vi "溶解氧电极校准.vi"() -> ()   [LabVIEW 2016, in "斯坦道多参数.lvlib"]
uses:
  <vilib>/Analysis/NI_AALBase.lvlib
  <vilib>/Utility/miscctls.llb/LVPointTypeDef.ctl
  <vilib>/Plasmionique/MB Master/MB_Master_Serial/MB_Master_Serial.lvclass
  C:/Program Files (x86)/National Instruments/LabVIEW 2016/vi.lib/Plasmionique/MB Master/MB_Master/MB_Master.lvclass
panel:
  out "变异系数":dbl
  out "standard deviation":dbl caption="标准差" format="%0.2f"
  out "mean":dbl caption="均值" format="%0.2f"
  out "测量读值":dbl
  out "偏移值补偿":dbl
  out "当前读值":dbl caption="饱和度值"
  out "提示":string
  in  "第二点通过校正":bool
  in  "第一点通过校正":bool
  in  "饱和度校正":bool
  in  "零点校正":bool
  out "气压补偿值":dbl
  out "盐度补偿值":dbl
  out "电极斜率":dbl
  out "电极零点":dbl
  # "溶解氧电极设定"
  # "%"
  # "ppt"
  # "%"
  # "hPa"
  # "%"
  # "mg/L"
  # "mg/L"
  # "电极校正"
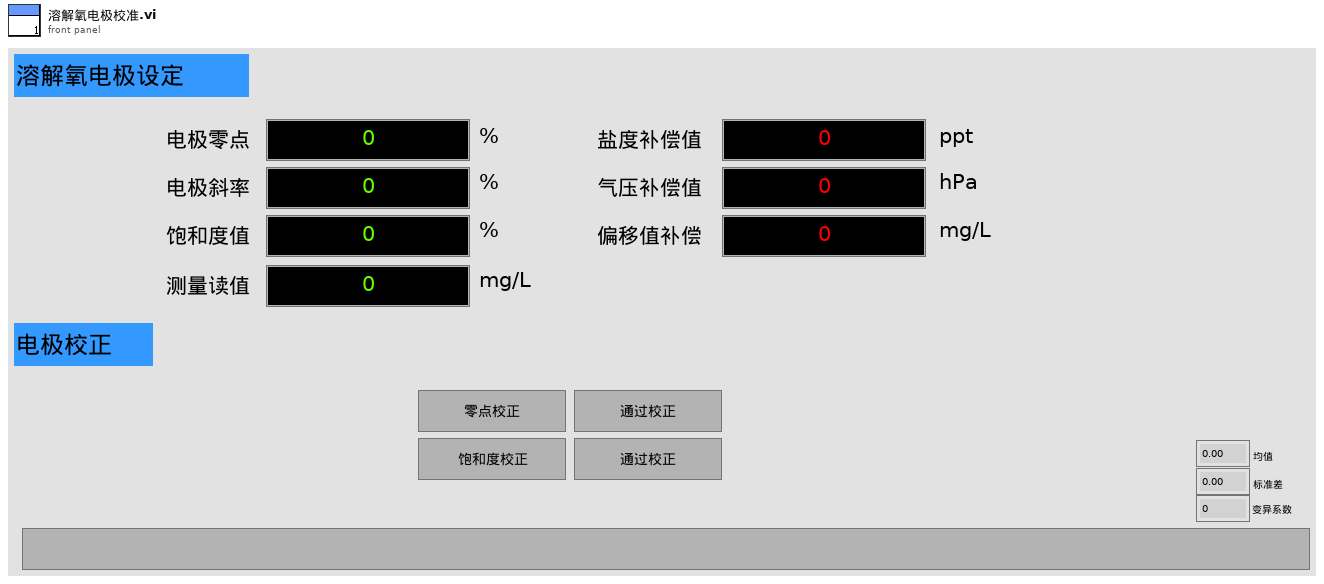
[diagram p1: front panel]
types:
  T1 = typedef "LVPointTypeDef.ctl" = cluster{"Horizontal":i16, "Vertical":i16}
  T2 = typedef "斯坦道多参数.lvlib/校准步骤.ctl" = enum16{"待机", "放置第一点标液", "第一点校准启动", "第一点校准写入", "第一点校准失败", "放置第二点标液", "第二点校准启动", "第二点校准写入", "第二点校准失败", "校准结果写入", "校准结束"}
  T3 = cluster{"电极状态标志":u16, "电极型号标志":u16, "溶解氧测量值":sgl, "温度测量值":sgl, "溶解氧饱和度值":sgl, "盐度补偿值":sgl, "大气压补偿值":sgl, "溶解氧偏移修正值":sgl, "温度偏移修正值":sgl, "手动温度补偿值":sgl, "溶解氧电极零点":sgl, "溶解氧电极斜率":sgl, "第1点标准值记录":sgl, "第1点信号值记录":sgl, "第1点温度值记录":sgl, "第2点标准值记录":sgl, "第2点信号值记录":sgl, "第2点温度值记录":sgl, "命令滤波设定":u16, "温度模式":enum16{"ATC", "MTC"}, "生产批次":u16, "电极序号":u16, "串口地址":u16, "串口波特率":enum16{"9600", "19200", "115200"}, "串口校验位":enum16{"NONE", "ODD", "EVEN"}, "串口停止位":enum16{"1bit", "2bit"}, "第一点标准值":sgl, "第二点标准值":sgl}
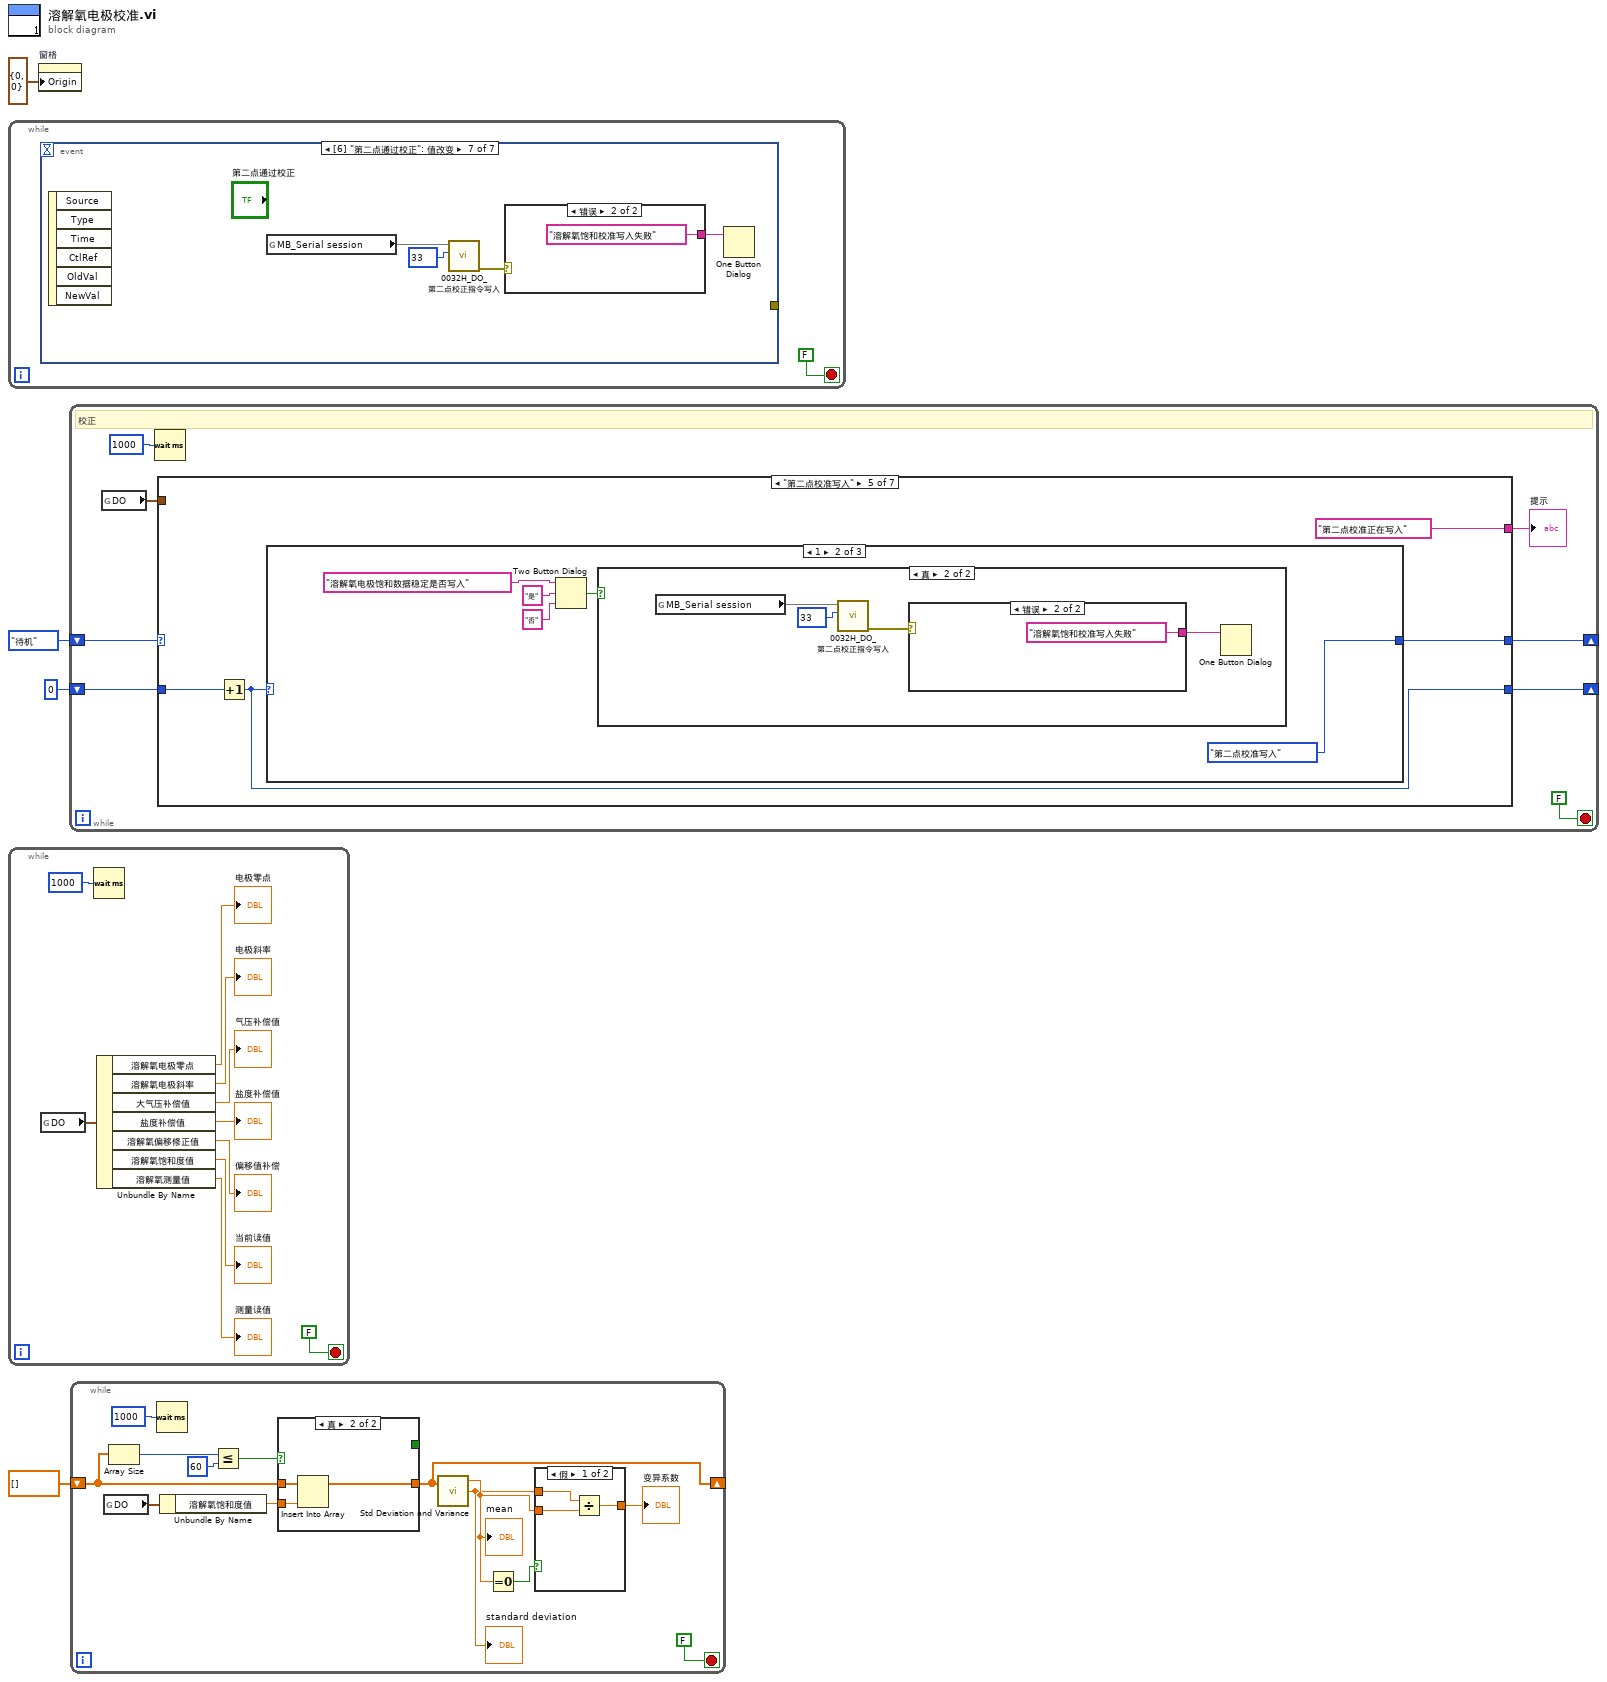
[diagram p0: block diagram]
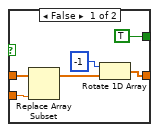
[diagram p3: hidden frame]
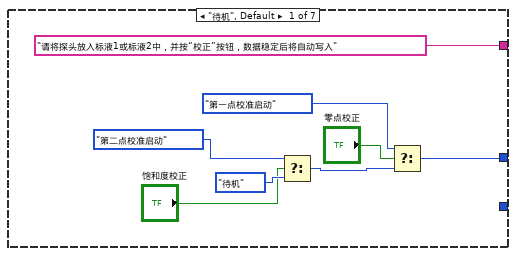
[diagram p4: hidden frame]
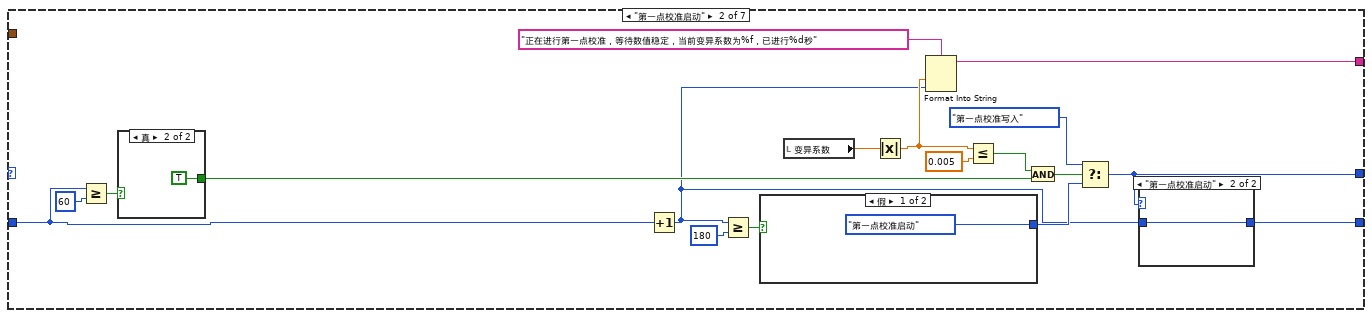
[diagram p5: hidden frame]
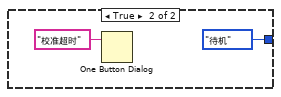
[diagram p7: hidden frame]
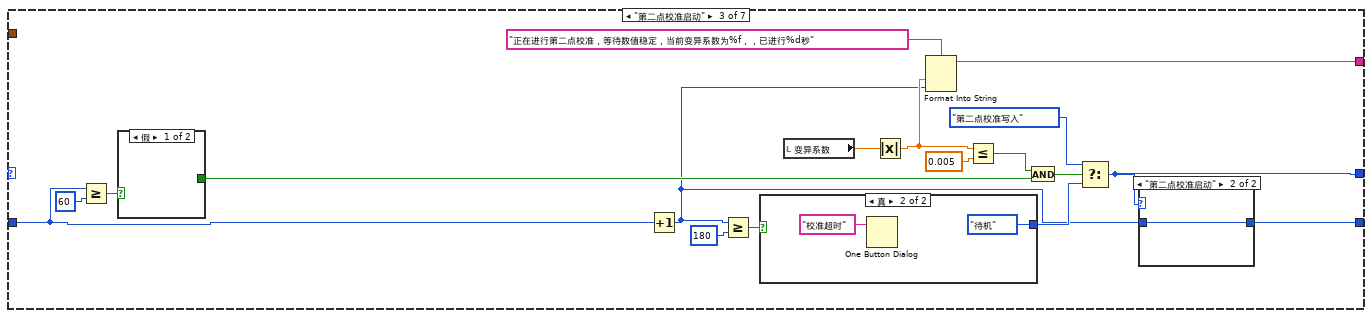
[diagram p9: hidden frame]
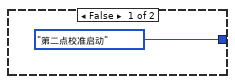
[diagram p11: hidden frame]
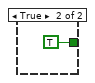
[diagram p12: hidden frame]
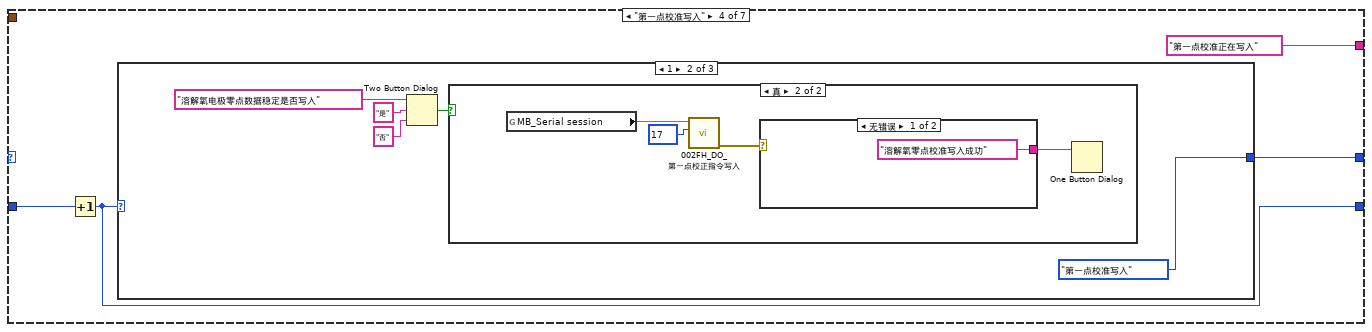
[diagram p13: hidden frame]
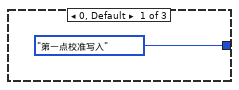
[diagram p14: hidden frame]
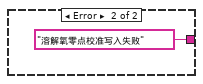
[diagram p16: hidden frame]
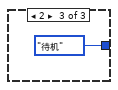
[diagram p17: hidden frame]
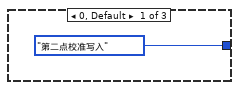
[diagram p18: hidden frame]
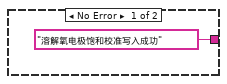
[diagram p20: hidden frame]
diagram:
  n1 = while {
    stop <- FALSE stop-if-true
    n2 = event shown="[6] \"第二点通过校正\": 值改变" {
      selector: _ -> [_ _ _ _ _ _ _]
      dyn-events: _ -> [_ _ _ _ _ _ _]
      timeout: _ -> [_ _ _ _ _ _ _]
      tunnel: [_ _ w10 w13 w16 _ _] -> _
      event Timeout {
        n3 = event-data() -> ()  [unwired: 1 in, 3 out]
      }
      event "盐度补偿值", "气压补偿值", "偏移值补偿": Mouse Down {
        n4 = event-data() -> ("CtlRef"=w7:refnum<vi>)  [unwired: 1 in, 7 out]
        n5 = property class="DigNum (严格)"(reference=w7) -> (reference out=w6:refnum<vi>, "Value"=w8:dbl)  [unwired: 1 in, 1 out]
        n6 = call "数字键盘.vi"("OldNumber"=w8) -> ("NewNumber"=w9:sgl)
        n7 = property class="DigNum (严格)"(reference=w6, "Val(Sgnl)"=w9) -> ()  [unwired: 1 in, 2 out]
      }
      event "盐度补偿值": Value Change {
        n8 = event-data() -> ("NewVal"=w11:dbl)  [unwired: 1 in, 5 out]
        n9 = global read "国弘过程全局变量.vi" "MB_Serial session"() -> (w12)
        n10 = call "0008H_DO_盐度补偿值写入.vi"("数值"=w11, "MB_Serial session in"=w12) -> ("error out"=w10:errorcluster)  [unwired: 8 in, 1 out]
      }
      event "气压补偿值": Value Change {
        n11 = event-data() -> ("NewVal"=w14:dbl)  [unwired: 1 in, 5 out]
        n12 = global read "国弘过程全局变量.vi" "MB_Serial session"() -> (w15)
        n13 = call "000AH_DO_大气压补偿值写入.vi"("数值"=w14, "MB_Serial session in"=w15) -> ("error out"=w13:errorcluster)  [unwired: 8 in, 1 out]
      }
      event "偏移值补偿": Value Change {
        n14 = event-data() -> ("NewVal"=w17:dbl)  [unwired: 1 in, 5 out]
        n15 = global read "国弘过程全局变量.vi" "MB_Serial session"() -> (w18)
        n16 = call "000CH_DO_DO偏移修正值写入.vi"("数值"=w17, "MB_Serial session in"=w18) -> ("error out"=w16:errorcluster)  [unwired: 8 in, 1 out]
      }
      event "第一点通过校正": Value Change {
        n17 = event-data() -> ()  [unwired: 1 in, 6 out]
        n18 = global read "国弘过程全局变量.vi" "MB_Serial session"() -> (w22)
        n19 = call "002FH_DO_第一点校正指令写入.vi"("数值"=u16 17, "MB_Serial session in"=w22) -> ("error out"=w19:errorcluster)  [unwired: 8 in, 1 out]
        n20 = case shown="无错误" w19 {
          tunnel: ["溶解氧零点校准写入成功" ("消息") "溶解氧零点校准写入失败" ("消息")] -> w20
          frame No Error {
          }
          frame Error {
          }
        }
        n21 = One Button Dialog(message=w20) -> ()  [unwired: 1 in, 1 out]
      }
      event "第二点通过校正": Value Change {
        n22 = event-data() -> ()  [unwired: 1 in, 6 out]
        n23 = global read "国弘过程全局变量.vi" "MB_Serial session"() -> (w27)
        n24 = call "0032H_DO_第二点校正指令写入.vi"("数值"=u16 33, "MB_Serial session in"=w27) -> ("error out"=w25:errorcluster)  [unwired: 8 in, 1 out]
        n25 = case shown="错误" w25 {
          tunnel: ["溶解氧电极饱和校准写入成功" ("消息") "溶解氧饱和校准写入失败" ("消息")] -> w26
          frame No Error {
          }
          frame Error {
          }
        }
        n26 = One Button Dialog(message=w26) -> ()  [unwired: 1 in, 1 out]
      }
    }
  }
  n27 = while {
    stop <- FALSE stop-if-true
    n28 = global read "国弘过程全局变量.vi" "DO"() -> (w38:T3)
    n29 = Wait (ms)(milliseconds to wait=u32 1000 ("等待时间（毫秒）")) -> ()  [unwired: 1 out]
    n30 = Unbundle By Name(w38) -> ("溶解氧电极零点"=→"电极零点":sgl, "溶解氧电极斜率"=→"电极斜率":sgl, "大气压补偿值"=→"气压补偿值":sgl, "盐度补偿值"=→"盐度补偿值":sgl, "溶解氧偏移修正值"=→"偏移值补偿":sgl, "溶解氧饱和度值"=→"当前读值":sgl, "溶解氧测量值"=→"测量读值":sgl)
  }
  n31 = property on="窗格" class="Pane"("Origin"=T1 {"Horizontal"=0, "Vertical"=0} ("原点")) -> ()  [unwired: 2 in, 2 out]
  n32 = while "While循环" {
    shift-right: [w47] -> _
    shift-left: 校准步骤."待机" ("枚举") -> [w48]
    shift-right: [w42] -> _
    shift-left: 0 -> [w43]
    stop <- FALSE stop-if-true
    # "校正"
    n33 = global read "国弘过程全局变量.vi" "DO"() -> (w45:T3)
    n34 = Wait (ms)(milliseconds to wait=u32 1000 ("等待时间（毫秒）")) -> ()  [unwired: 1 out]
    n35 = case shown="\"第二点校准写入\"" w48 {
      tunnel: [w55 w61 w84 w103 w120 校准步骤."待机" ("枚举") 校准步骤."待机" ("枚举")] -> w47
      tunnel: ["请将探头放入标液1或标液2中，并按“校正”按钮，数据稳定后将自动写入" ("提示") w71 w89 "第一点校准正在写入" ("提示") "第二点校准正在写入" ("提示") "第一点校准失败" ("提示") "第二点校准失败" ("提示")] -> w41
      tunnel: w45 -> [_ _ _ _ _ _ _]
      tunnel: w43 -> [_ w58 w80 w105 w122 w138 w143]
      tunnel: [_ w59 w82 w104 w121 w137 w142] -> w42
      frame "待机", Default {
        n36 = Select(t=校准步骤."第二点校准启动" ("枚举"), s="饱和度校正", f=校准步骤."待机" ("枚举")) -> (s? t:f=w51:T2)
        n37 = Select(t=校准步骤."第一点校准启动" ("枚举"), s="零点校正", f=w51) -> (s? t:f=w55:T2)
      }
      frame "第一点校准启动" {
        n38 = Greater Or Equal?(x=w58, y=60) -> (x >= y?=w73:bool)
        n39 = case shown="真" w73 {
          tunnel: [_ TRUE] -> w68
          frame False {
          }
          frame True {
          }
        }
        n40 = Increment(x=w58) -> (x+1=w60:i32)
        n41 = Greater Or Equal?(x=w60, y=180) -> (x >= y?=w63:bool)
        n42 = case shown="假" w63 {
          tunnel: [校准步骤."第一点校准启动" ("枚举") 校准步骤."待机" ("枚举")] -> w62
          frame False {
          }
          frame True {
            n43 = One Button Dialog(message="校准超时" ("消息")) -> ()  [unwired: 1 in, 1 out]
          }
        }
        n44 = local read "变异系数"() -> (w57:dbl)
        n45 = Absolute Value(x=w57) -> (abs(x)=w65:dbl)
        n46 = Format Into String(format string="正在进行第一点校准，等待数值稳定，当前变异系数为%f，已进行%d秒" ("格式字符串"), w65, w60) -> (resulting string=w71:string)  [unwired: 2 in, 1 out]
        n47 = Less Or Equal?(x=w65, y=0.005) -> (x <= y?=w67:bool)
        n48 = And(x=w67, y=w68) -> (x .and. y?=w66:bool)
        n49 = Select(t=校准步骤."第一点校准写入" ("枚举"), s=w66, f=w62) -> (s? t:f=w61:T2)
        n50 = case shown="\"第一点校准启动\"" w61 {
          tunnel: w60 -> [_ w75]
          tunnel: [_ w75] -> w59
          frame "待机", Default {
          }
          frame "第一点校准启动" {
          }
        }
      }
      frame "第二点校准启动" {
        n51 = Greater Or Equal?(x=w80, y=60) -> (x >= y?=w96:bool)
        n52 = case shown="假" w96 {
          tunnel: [_ TRUE] -> w92
          frame False {
          }
          frame True {
          }
        }
        n53 = Increment(x=w80) -> (x+1=w83:i32)
        n54 = Greater Or Equal?(x=w83, y=180) -> (x >= y?=w86:bool)
        n55 = case shown="真" w86 {
          tunnel: [校准步骤."第二点校准启动" ("枚举") 校准步骤."待机" ("枚举")] -> w85
          frame False {
          }
          frame True {
            n56 = One Button Dialog(message="校准超时" ("消息")) -> ()  [unwired: 1 in, 1 out]
          }
        }
        n57 = local read "变异系数"() -> (w81:dbl)
        n58 = Absolute Value(x=w81) -> (abs(x)=w88:dbl)
        n59 = Format Into String(format string="正在进行第二点校准，等待数值稳定，当前变异系数为%f，，已进行%d秒" ("格式字符串"), w88, w83) -> (resulting string=w89:string)  [unwired: 2 in, 1 out]
        n60 = Less Or Equal?(x=w88, y=0.005) -> (x <= y?=w91:bool)
        n61 = And(x=w91, y=w92) -> (x .and. y?=w90:bool)
        n62 = Select(t=校准步骤."第二点校准写入" ("枚举"), s=w90, f=w85) -> (s? t:f=w84:T2)
        n63 = case shown="\"第二点校准启动\"" w84 {
          tunnel: w83 -> [_ w98]
          tunnel: [_ w98] -> w82
          frame "待机", Default {
          }
          frame "第二点校准启动" {
          }
        }
      }
      frame "第一点校准写入" {
        n64 = Increment(x=w105) -> (x+1=w104:i32)
        n65 = case shown="1" w104 {
          tunnel: [校准步骤."第一点校准写入" ("枚举") 校准步骤."第一点校准写入" ("枚举") 校准步骤."待机" ("枚举")] -> w103
          frame 0, Default {
          }
          frame 1 {
            n66 = Two Button Dialog(message="溶解氧电极零点数据稳定是否写入" ("消息"), 1:"否" ("F按钮名称（“取消”）"), 2:"是" ("T按钮名称（“确定”）")) -> (T button?=w108:bool)
            n67 = case shown="真" w108 {
              frame False {
              }
              frame True {
                n68 = global read "国弘过程全局变量.vi" "MB_Serial session"() -> (w115)
                n69 = call "002FH_DO_第一点校正指令写入.vi"("数值"=u16 17, "MB_Serial session in"=w115) -> ("error out"=w113:errorcluster)  [unwired: 8 in, 1 out]
                n70 = case shown="无错误" w113 {
                  tunnel: ["溶解氧零点校准写入成功" ("消息") "溶解氧零点校准写入失败" ("消息")] -> w114
                  frame No Error {
                  }
                  frame Error {
                  }
                }
                n71 = One Button Dialog(message=w114) -> ()  [unwired: 1 in, 1 out]
              }
            }
          }
          frame 2 {
          }
        }
      }
      frame "第二点校准写入" {
        n72 = Increment(x=w122) -> (x+1=w121:i32)
        n73 = case shown="1" w121 {
          tunnel: [校准步骤."第二点校准写入" ("枚举") 校准步骤."第二点校准写入" ("枚举") 校准步骤."待机" ("枚举")] -> w120
          frame 0, Default {
          }
          frame 1 {
            n74 = Two Button Dialog(message="溶解氧电极饱和数据稳定是否写入" ("消息"), 1:"否" ("F按钮名称（“取消”）"), 2:"是" ("T按钮名称（“确定”）")) -> (T button?=w125:bool)
            n75 = case shown="真" w125 {
              frame False {
              }
              frame True {
                n76 = global read "国弘过程全局变量.vi" "MB_Serial session"() -> (w133)
                n77 = call "0032H_DO_第二点校正指令写入.vi"("数值"=u16 33, "MB_Serial session in"=w133) -> ("error out"=w130:errorcluster)  [unwired: 8 in, 1 out]
                n78 = case shown="错误" w130 {
                  tunnel: ["溶解氧电极饱和校准写入成功" ("消息") "溶解氧饱和校准写入失败" ("消息")] -> w131
                  frame No Error {
                  }
                  frame Error {
                  }
                }
                n79 = One Button Dialog(message=w131) -> ()  [unwired: 1 in, 1 out]
              }
            }
          }
          frame 2 {
          }
        }
      }
      frame "第一点校准失败" {
        n80 = Two Button Dialog(message="第一点校准失败是否重新校准" ("消息")) -> ()  [unwired: 2 in, 1 out]
        n81 = Increment(x=w138) -> (x+1=w137:i32)
      }
      frame "第二点校准失败" {
        n82 = Increment(x=w143) -> (x+1=w142:i32)
      }
    }
    "提示" <- w41
  }
  n83 = while {
    shift-right: [w151] -> _
    shift-left: sgl[] [] -> [w154]
    stop <- FALSE stop-if-true
    n84 = global read "国弘过程全局变量.vi" "DO"() -> (w148:T3)
    n85 = Array Size(array=w154) -> (size(s)=w156:i32)
    n86 = Wait (ms)(milliseconds to wait=u32 1000 ("等待时间（毫秒）")) -> ()  [unwired: 1 out]
    n87 = Unbundle By Name(w148) -> ("溶解氧饱和度值"=w153:sgl)
    n88 = Less Or Equal?(x=w156, y=60) -> (x <= y?=w155:bool)
    n89 = case shown="真" w155 {
      tunnel: w154 -> [w167 w170]
      tunnel: w153 -> [w165 w169]
      tunnel: [w163 w168] -> w151
      tunnel: [TRUE _] -> _
      frame False {
        n90 = Replace Array Subset(array=w167, new element=w165) -> (w166:sgl[])  [unwired: 1 in]
        n91 = Rotate 1D Array(1:w166, 2:-1 ("n")) -> (0:w163:sgl[])
      }
      frame True {
        n92 = Insert Into Array(array=w170, new element=w169) -> (w168:sgl[])  [unwired: 1 in]
      }
    }
    n93 = call <vilib>:"Std Deviation and Variance.vi"("X"=w151) -> ("mean"=w147:dbl, "standard deviation"=w146:dbl)  [unwired: 1 in, 1 out]
    "mean" <- w147
    "standard deviation" <- w146
    n94 = Equal To 0?(x=w147) -> (x = 0?=w152:bool)
    n95 = case shown="假" w152 {
      tunnel: w146 -> [w161 _]
      tunnel: [w160 _] -> w150
      tunnel: w147 -> [w159 _]
      frame False {
        n96 = Divide(x=w161, y=w159) -> (x/y=w160:dbl)
      }
      frame True {
      }
    }
    "变异系数" <- w150
  }
